vi "fn.detedge-fall.vi"(3 "Signal in":bool) -> (0 "Signal out":bool, 1 "Edge?":bool)   [LabVIEW 2019]
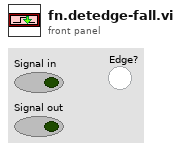
[diagram p1: front panel]
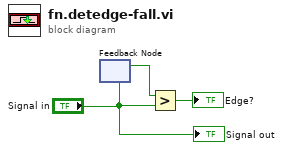
[diagram p0: block diagram]
diagram:
  n1 = feedback #1() -> (w3:bool)  [unwired: 1 in]
  n2 = feedback-in #1("Signal in") -> ()
  n3 = Greater?(x=w3, y="Signal in") -> (0:→"Edge?":bool)
  "Signal out" <- "Signal in"
